vi "build.elementToParamString.vi"(11 "UiStepFunction":T1) -> (2 "params":string[](array[string]), 3 "source":string)   [LabVIEW 2024]
uses:
  controls/type.step-builder.ctl
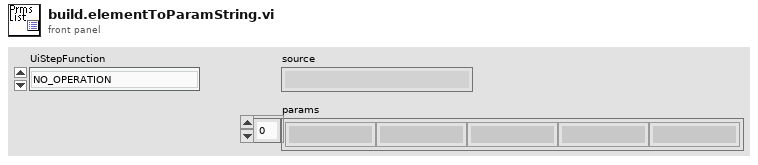
[diagram p1: front panel]
types:
  T1 = typedef "type.step-builder.ctl" = enum16{"NO_OPERATION", "DELAY-JUMP", "DELAY", "JUMP", "COMPLETE", "SCHEDULER", "IRR-CHECK", "UNIT-CHECK", "UNIT-SAMPLE", "UNIT-DOSE", "LOG-REPORT", "LOG-MESSAGE", "IO-READ", "IO-READ-MANY", "IO-WRITE", "IO-COMPARE-OUT", "IO-COMPARE-IN", "PROC-START", "PROC-STOP", "PROC-LOAD", "PROC-IS-COMPLETED", "RECORD-MOVE", "GET-RH", "GET-UV", "GET-WD", "GET-WS", "OCS-CHECK", "OCS-RECORD"}
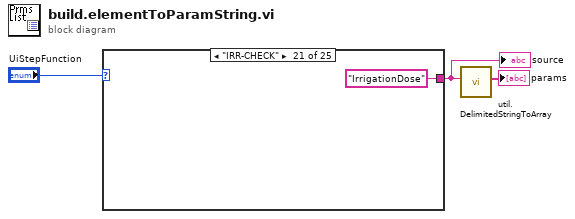
[diagram p0: block diagram]
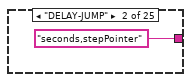
[diagram p3: hidden frame]
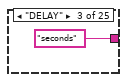
[diagram p4: hidden frame]
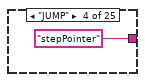
[diagram p5: hidden frame]
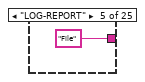
[diagram p6: hidden frame]
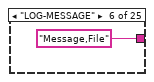
[diagram p7: hidden frame]
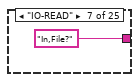
[diagram p8: hidden frame]
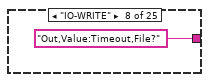
[diagram p9: hidden frame]
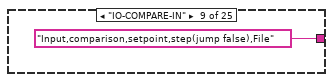
[diagram p10: hidden frame]
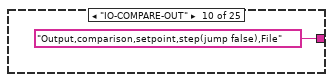
[diagram p11: hidden frame]
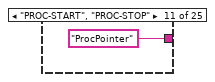
[diagram p12: hidden frame]
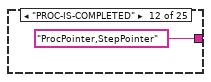
[diagram p13: hidden frame]
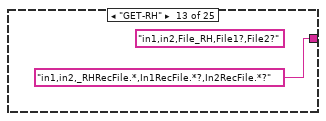
[diagram p14: hidden frame]
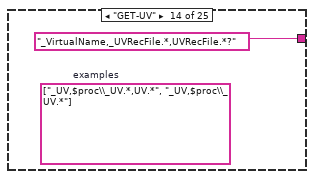
[diagram p15: hidden frame]
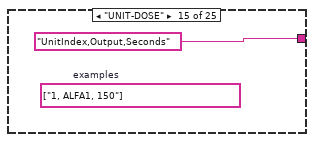
[diagram p16: hidden frame]
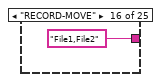
[diagram p17: hidden frame]
diagram:
  n1 = case shown="\"IRR-CHECK\"" "UiStepFunction" {
    tunnel: [_ "seconds,stepPointer" ("parameters") "seconds" ("source") "stepPointer" ("source") "File" ("source") "Message,File" ("source") "In,File?" ("source") "Out,Value:Timeout,File?" ("source") "Input,comparison,setpoint,step(jump false),File" ("source") "Output,comparison,setpoint,step(jump false),File" ("source") "ProcPointer" ("source") "ProcPointer,StepPointer" ("source") "in1,in2,_RHRecFile.*,In1RecFile.*?,In2RecFile.*?" ("source") "_VirtualName,_UVRecFile.*,UVRecFile.*?" ("source") "UnitIndex,Output,Seconds" ("source") "File1,File2" ("source") _ _ _ _ "IrrigationDose" ("source") _ _ _ _] -> w2
    frame "NO_OPERATION", Default {
    }
    frame "DELAY-JUMP" {
    }
    frame "DELAY" {
    }
    frame "JUMP" {
    }
    frame "LOG-REPORT" {
    }
    frame "LOG-MESSAGE" {
    }
    frame "IO-READ" {
    }
    frame "IO-WRITE" {
    }
    frame "IO-COMPARE-IN" {
    }
    frame "IO-COMPARE-OUT" {
    }
    frame "PROC-START", "PROC-STOP" {
    }
    frame "PROC-IS-COMPLETED" {
    }
    frame "GET-RH" {
      (unwired) "in1,in2,File_RH,File1?,File2?" ("source")
    }
    frame "GET-UV" {
      (unwired) string[] ["_UV,$proc\\_UV.*,UV.*", "_UV,$proc\\_UV.*"]  # examples
    }
    frame "UNIT-DOSE" {
      (unwired) string[] ["1, ALFA1, 150"]  # examples
    }
    frame "RECORD-MOVE" {
    }
    frame "GET-WD" {
    }
    frame "GET-WS" {
    }
    frame "OCS-CHECK" {
    }
    frame "SCHEDULER" {
    }
    frame "IRR-CHECK" {
    }
    frame "UNIT-CHECK" {
    }
    frame "UNIT-SAMPLE" {
    }
    frame "IO-READ-MANY" {
    }
    frame "PROC-LOAD" {
    }
  }
  "source" <- w2
  n2 = call "util.DelimitedStringToArray.vi"("delimitaed string"=w2) -> ("array out"=→"params":string[])  [unwired: 10 in]
